vi "SetROI.vi"(8 "error in (no error)":errorcluster, 10 "Setting.ROI":T1, 11 "Camera_Prime95B in":refnum<class "Camera_Prime95B.lvclass">) -> (0 "error out":errorcluster, 3 "Camera_Prime95B out":refnum<class "Camera_Prime95B.lvclass">)   [LabVIEW 2020, in "Camera_Prime95B.lvlib" / "Camera_Prime95B.lvclass"]
uses:
  Camera_Prime95B.lvclass
  Camera_Prime95B.lvclass/Camera_Prime95B.ctl
  E:/Development/DevHardSoftware/MMicroscopyAF/Model/Real Hardware/Camera_Prime95B/Camera_Prime95B/Dependencies/PVCamNET.dll
  Dependencies/PVCamNET.dll
  HAL Layer/Component/Camera/Camera/Camera.lvclass
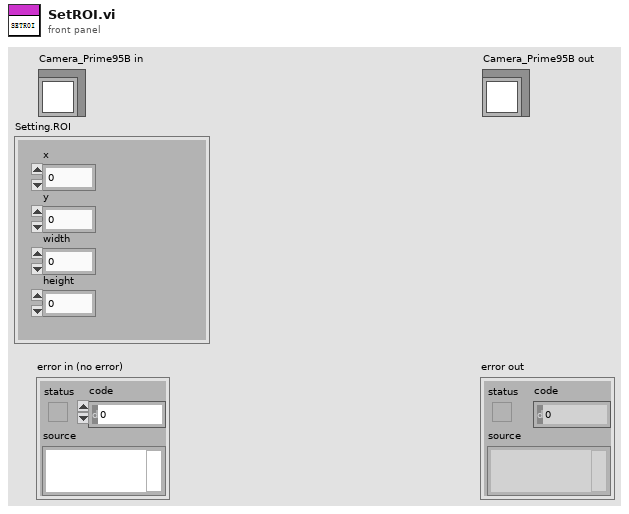
[diagram p1: front panel]
types:
  T1 = cluster{"x":dbl, "y":dbl, "width":dbl, "height":dbl}
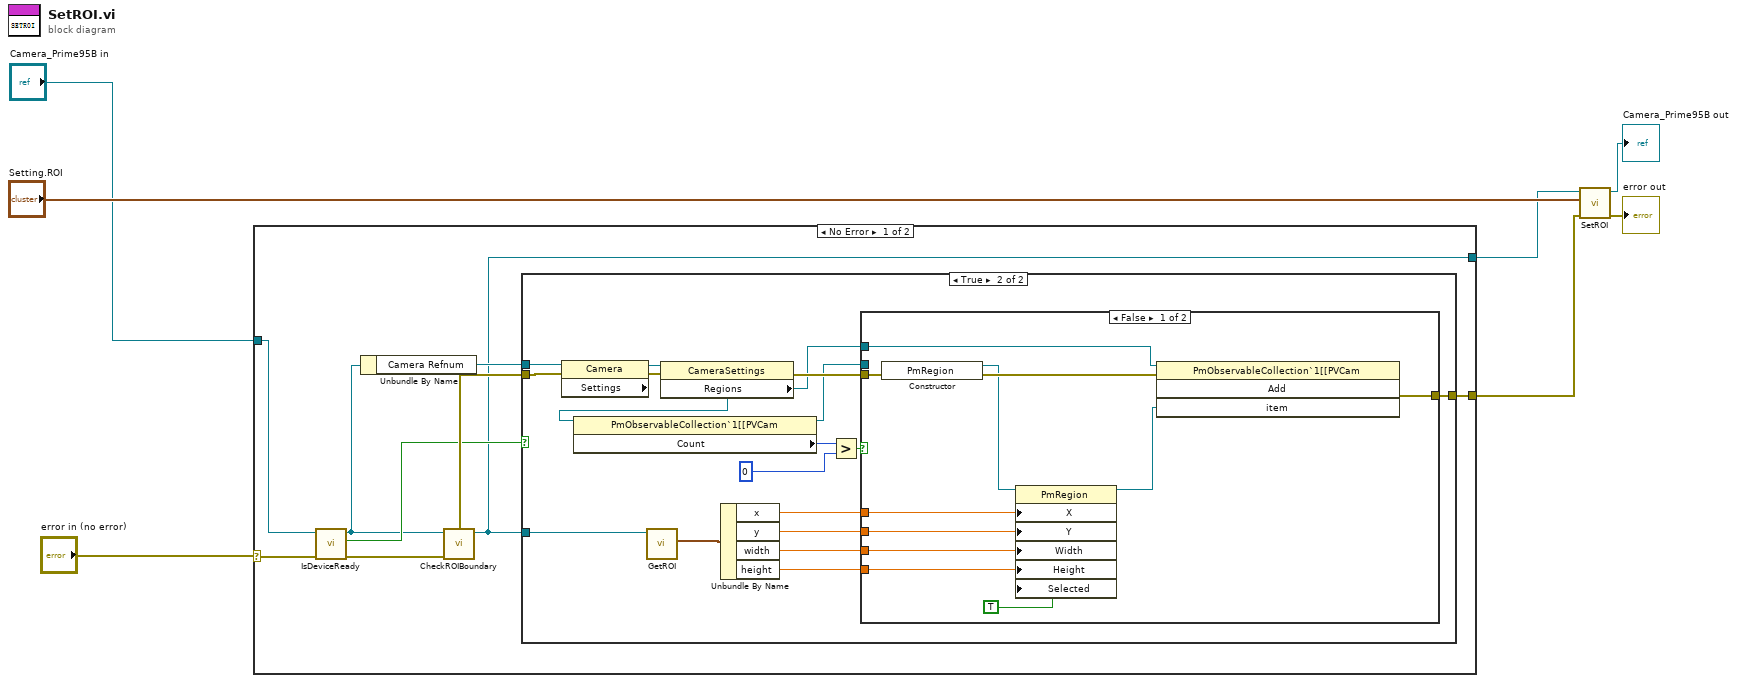
[diagram p0: block diagram]
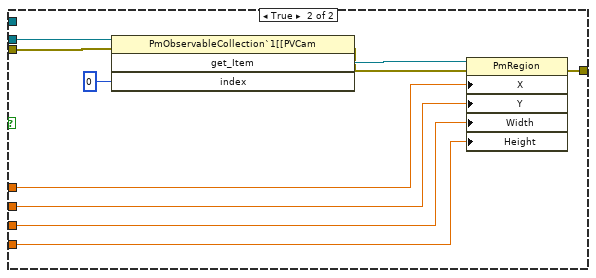
[diagram p3: hidden frame]
diagram:
  n1 = case shown="No Error" "error in (no error)" {
    selector: "error in (no error)" -> [w14 w57]
    tunnel: [w16 w57] -> w1
    tunnel: "Camera_Prime95B in" -> [w13 w56]
    tunnel: [w8 w56] -> w2
    frame No Error {
      n2 = call-dynamic "IsDeviceReady.vi"("error in (no error)"=w14, "Camera_Prime95B in"=w13) -> ("error out"=w9:errorcluster, "Ready?"=w12:bool, "Camera_Prime95B out"=w10:refnum<class "Camera_Prime95B.lvclass">)  [unwired: 7 in]
      n3 = Unbundle By Name(w10) -> ("Camera Refnum"=w11:refnum<k24>)
      n4 = call-dynamic "CheckROIBoundary.vi"("error in (no error)"=w9, "Camera in"=w10) -> ("error out"=w15:errorcluster, "Camera out"=w8:refnum<class "Camera_Prime95B.lvclass">)  [unwired: 7 in, 1 out]
      n5 = case shown="True" w12 {
        tunnel: [w17 w21] -> w16
        tunnel: w15 -> [w17 w32]
        tunnel: w11 -> [_ w19]
        tunnel: w8 -> [_ w18]
        frame False {
        }
        frame True {
          n6 = property class="Camera"(reference=w19, error in=w32) -> (error out=w33:errorcluster, "Settings"=w34:refnum<k24>)  [unwired: 1 out]
          n7 = call-dynamic "GetROI.vi"("Camera in"=w18) -> ("Setting.ROI"=w26:T1)  [unwired: 8 in, 2 out]
          n8 = property class="CameraSettings"(reference=w34, error in=w33) -> (error out=w28:errorcluster, "Regions"=w20:refnum<k24>)  [unwired: 1 out]
          n9 = property class="PmObservableCollection`1[[PVCam"(reference=w20) -> (reference out=w27:refnum<k24>, "Count"=w31:i32)  [unwired: 1 in, 1 out]
          n10 = Unbundle By Name(w26) -> ("x"=w25:dbl, "y"=w24:dbl, "width"=w23:dbl, "height"=w22:dbl)
          n11 = Greater?(x=w31, y=0) -> (0:w30:bool)
          n12 = case shown="False" w30 {
            tunnel: w27 -> [_ w53]
            tunnel: w28 -> [w42 w52]
            tunnel: [w45 w50] -> w21
            tunnel: w25 -> [w39 w49]
            tunnel: w24 -> [w38 w48]
            tunnel: w23 -> [w37 w47]
            tunnel: w22 -> [w36 w46]
            tunnel: w20 -> [w35 _]
            frame False {
              n13 = constructor class="PmRegion"(error in=w42) -> (reference out=w40:refnum<k24>, error out=w41:errorcluster)  [unwired: 2 in, 1 out]
              n14 = property class="PmRegion"(reference=w40, "X"=w39, "Y"=w38, "Width"=w37, "Height"=w36, "Selected"=TRUE) -> (reference out=w44:refnum<k24>)  [unwired: 1 in, 1 out]
              n15 = invoke class="PmObservableCollection`1[[PVCam" method="Add"(reference=w35, error in=w41, "item"=w44) -> (error out=w45:errorcluster)  [unwired: 1 in, 3 out]
            }
            frame True {
              n16 = invoke class="PmObservableCollection`1[[PVCam" method="get_Item"(reference=w53, error in=w52, "index"=0) -> (error out=w51:errorcluster, "get_Item"=w55:refnum<k24>)  [unwired: 1 in, 2 out]
              n17 = property class="PmRegion"(reference=w55, error in=w51, "X"=w49, "Y"=w48, "Width"=w47, "Height"=w46) -> (error out=w50:errorcluster)  [unwired: 1 out]
            }
          }
        }
      }
    }
    frame Error {
    }
  }
  n18 = call-parent "SetROI.vi"("error in (no error)"=w1, "Setting.ROI"="Setting.ROI", "Camera in"=w2) -> ("error out"=→"error out":errorcluster, "Camera out"=→"Camera_Prime95B out":refnum<class "Camera_Prime95B.lvclass">)  [unwired: 7 in]
